vi "Case Selector.vi"(9 "Click Down":bool, 10 "Click Up":bool, 11 "Dump All?":bool) -> (1 "Down Pressed?":bool, 2 "Up Pressed?":bool, 3 "State":i32)   [LabVIEW 2015]
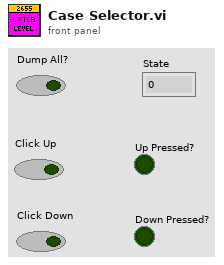
[diagram p1: front panel]
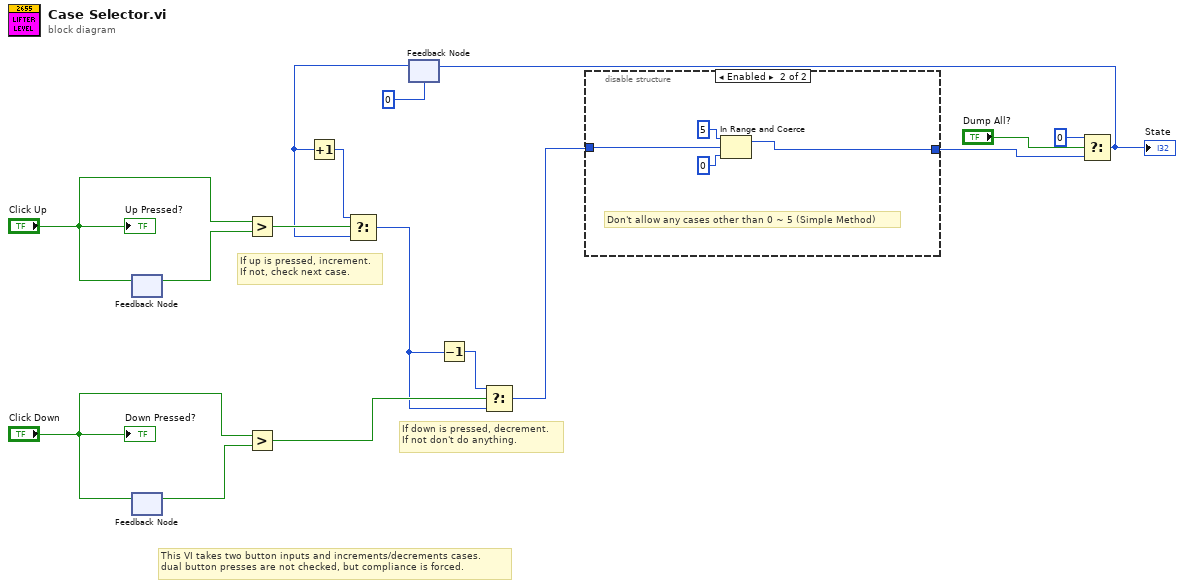
[diagram p0: block diagram]
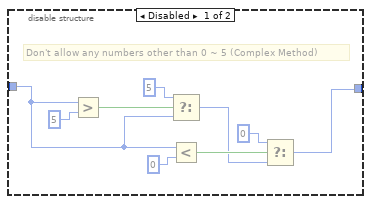
[diagram p2: hidden frame]
diagram:
  # "If down is pressed, decrement.\nIf not don't do anything."
  # "If up is pressed, increment.\nIf not, check next case."
  # "This VI takes two button inputs and increments/decrements cases.\ndual button presses are not checked, but compliance is forced."
  n1 = feedback #1() -> (w15:bool)  [unwired: 1 in]
  n2 = feedback-in #1("Click Up") -> ()
  n3 = feedback #2() -> (w13:bool)  [unwired: 1 in]
  n4 = feedback-in #2("Click Down") -> ()
  n5 = Greater?(x="Click Up", y=w15) -> (0:w12:bool)
  n6 = Greater?(x="Click Down", y=w13) -> (0:w11:bool)
  n7 = feedback #3(0) -> (w8:i32)
  n8 = Increment(x=w8) -> (x+1=w7:i32)
  n9 = Select(t=w7, s=w12, f=w8) -> (s? t:f=w10:i32)
  n10 = Decrement(x=w10) -> (x-1=w9:i32)
  n11 = Select(t=w9, s=w11, f=w10) -> (s? t:f=w6:i32)
  n12 = disable-structure shown="Enabled" {
    disable-tunnel: [w24 w26] -> w4
    disable-tunnel: w6 -> [w17 w29]
    frame Disabled {
      # "Don't allow any numbers other than 0 ~ 5 (Complex Method)"
      n13 = Greater?(x=w17, y=5) -> (0:w19:bool)
      n14 = Select(t=5, s=w19, f=w17) -> (s? t:f=w20:i32)
      n15 = Less?(x=w17, y=0) -> (x < y?=w22:bool)
      n16 = Select(t=0, s=w22, f=w20) -> (s? t:f=w24:i32)
    }
    frame Enabled {
      # "Don't allow any cases other than 0 ~ 5 (Simple Method)"
      n17 = In Range and Coerce(upper limit=5, x=w29, lower limit=0) -> (coerced(x)=w26:i32)  [unwired: 1 out]
    }
  }
  n18 = Select(t=0, s="Dump All?", f=w4) -> (s? t:f=w1:i32)
  "State" <- w1
  n19 = feedback-in #3(w1) -> ()
  "Down Pressed?" <- "Click Down"
  "Up Pressed?" <- "Click Up"
